vi "Random Cell Address.vi"() -> (3 "Random Cell Address":string)   [LabVIEW 2020, in "Test Open Xml.lvclass"]
uses:
  Test Open Xml.lvclass
  <vilib>/numeric/Random Number (Range) U64.vi
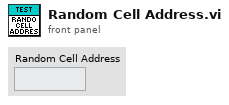
[diagram p1: front panel]
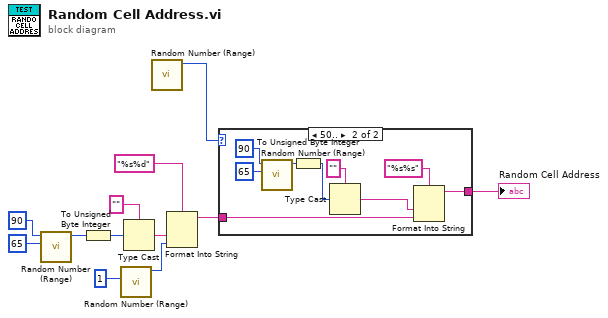
[diagram p0: block diagram]
diagram:
  n1 = call-poly <vilib>:"Random Number (Range).vi"("lower bound (0)"=u64 65, "upper bound (100)"=u64 90) -> ("number"=w11:u64)  [unwired: 9 in]
  n2 = To Unsigned Byte Integer(number=w11) -> (unsigned 8bit integer=w1:u8)
  n3 = call-poly <vilib>:"Random Number (Range).vi"("lower bound (0)"=u64 1) -> ("number"=w6:u64)  [unwired: 10 in]
  n4 = Type Cast(type="", x=w1) -> (*(type *) &x=w7:string)
  n5 = call-poly <vilib>:"Random Number (Range).vi"() -> ("number"=w2:u64)  [unwired: 11 in]
  n6 = Format Into String(format string="%s%d", w7, w6) -> (resulting string=w3:string)  [unwired: 2 in, 1 out]
  n7 = case shown="50.." w2 {
    tunnel: [w13 w22] -> w4
    tunnel: w3 -> [w13 w20]
    frame 0, Default {
    }
    frame 50.. {
      n8 = call-poly <vilib>:"Random Number (Range).vi"("lower bound (0)"=u64 65, "upper bound (100)"=u64 90) -> ("number"=w15:u64)  [unwired: 9 in]
      n9 = To Unsigned Byte Integer(number=w15) -> (unsigned 8bit integer=w14:u8)
      n10 = Type Cast(type="", x=w14) -> (*(type *) &x=w18:string)
      n11 = Format Into String(format string="%s%s", w18, w20) -> (resulting string=w22:string)  [unwired: 2 in, 1 out]
    }
  }
  "Random Cell Address" <- w4
